vi "DroneCascadePhotos.vi"() -> ()   [LabVIEW 2017]
uses:
  <vilib>/LVH/AR Drone Toolkit/Decode NavData/Typedefs/NavData Demo.ctl
  <vilib>/LVH/AR Drone Toolkit/AR Drone.lvlib
panel:
  out "Photos Taken":dbl
  in  "Take Photos":bool
  in  "Setup Parameters":T1={"Drone IP address"="192.168.1.1", "Home IP address"="192.168.1.2", "Flight Mode"=enum."INDOOR MODE", "Mounted Hull"=enum."INDOOR HULL", "Video Camera"=2, "Max Altitude (m)"=3.0, "Max Pitch and Roll Angle (deg)"=10.0, "Max Vertical Speed (m/s)"=0.7, "Max Yaw Speed (deg/s)"=100.0} {"Video Camera" items=["Bottom Camera"=1, "Front Camera"=0, "Front in Bottom"=3, "Bottom in Front"=2]}
  out "Video Stream":picture
  out "NavData Out":T2
  out "Battery Remaining":dbl(slide) scale=0.0..100.0
  in  "Hover":bool
  in  "Take Off/Land":bool
  in  "Emergency Landing":bool
  in  "stop 2":bool
  in  "Control Cluster":T3 {"Yaw Speed" scale=-1.0..1.0; "Vertical Speed" scale=-1.0..1.0; "Pitch" scale=-1.0..1.0; "Roll" scale=-1.0..1.0}
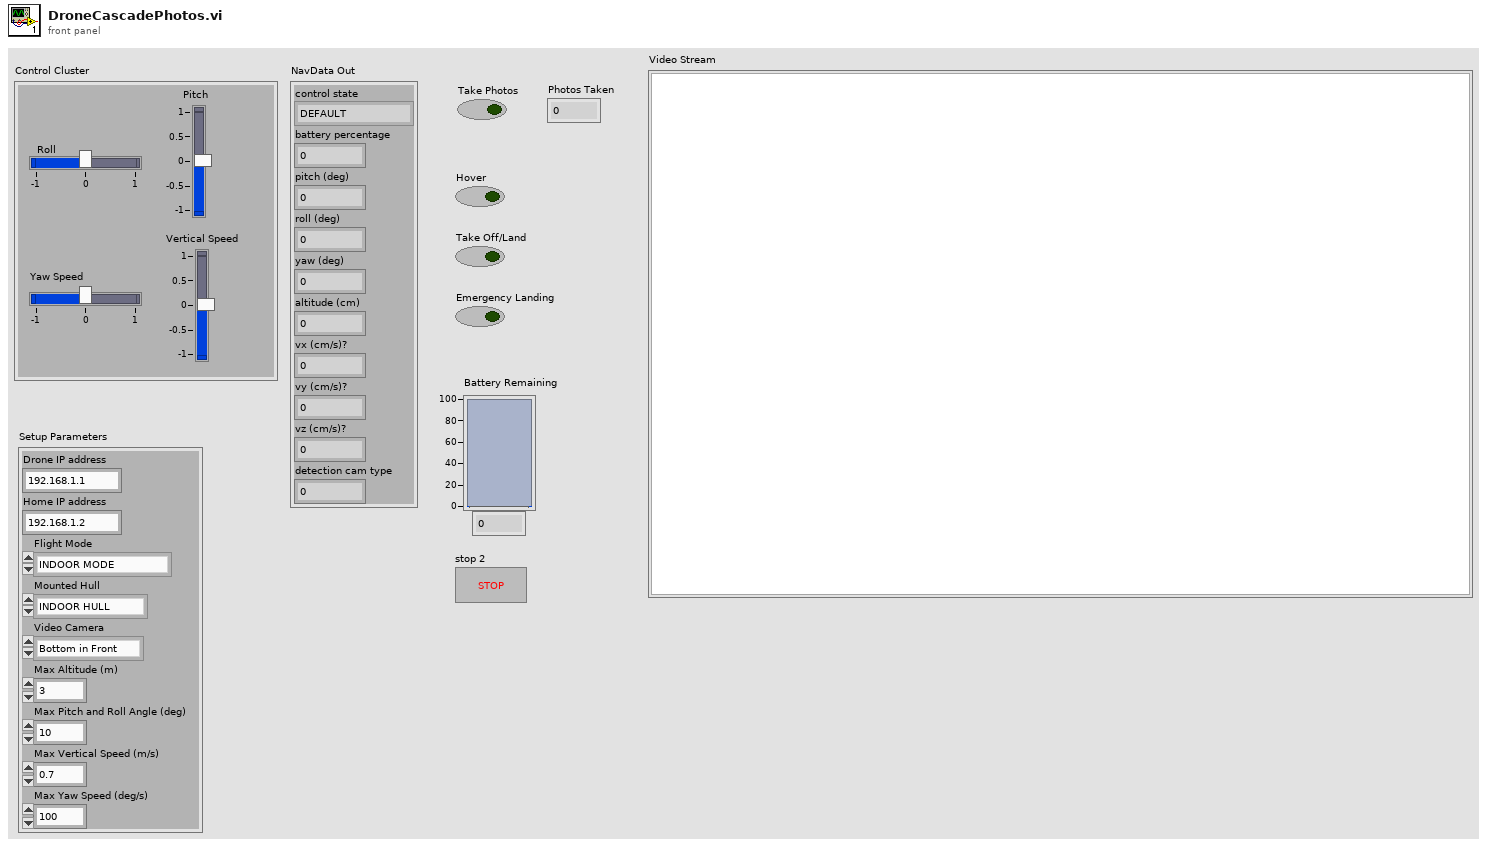
[diagram p1: front panel]
types:
  T1 = cluster{"Drone IP address":string, "Home IP address":string, "Flight Mode":enum8{"OUTDOOR MODE", "INDOOR MODE"}, "Mounted Hull":enum8{"OUTDOOR HULL", "INDOOR HULL"}, "Video Camera":u8, "Max Altitude (m)":sgl, "Max Pitch and Roll Angle (deg)":sgl, "Max Vertical Speed (m/s)":sgl, "Max Yaw Speed (deg/s)":sgl}
  T2 = typedef "AR Drone.lvlib/NavData Demo.ctl" = cluster{"control state":enum32{"DEFAULT", "INIT", "LANDING", "FLYING", "HOVERING", "TEST", "TRANS_TAKEOFF", "TRANS_GOTOFIX", "TRANS_LANDING"}, "battery percentage":u32, "pitch (deg)":sgl, "roll (deg)":sgl, "yaw (deg)":sgl, "altitude (cm)":u32, "vx (cm/s)?":sgl, "vy (cm/s)?":sgl, "vz (cm/s)?":sgl, "detection cam type":u32}
  T3 = cluster{"Roll":sgl, "Pitch":sgl, "Vertical Speed":sgl, "Yaw Speed":sgl}
  T4 = typedef "AR Drone.lvlib/AR Drone Resource.ctl" = cluster{"UDP Control Connection":refnum<k16>, "UDP NavData Connection":refnum<k16>, "UDP Video Connection (Drone 1.0)":refnum<k16>, "TCP Video Connection (Drone 2.0)":refnum<k5>, "TCP Control Port Connection":refnum<k5>, "Drone IP address":string, "Drone Command Port":u16, "Drone NavData Port":u16, "Drone Vid Stream Port":u16, "Drone TCP Control Port":u16, "Home IP address":string, "Home Command Port":u16, "Home NavData Port":u16, "Home Vid Stream Port":u16, "Drone Version":i32, "Drone Index":dbl}
  T5 = typedef "IMAQ Image.ctl" = refnum<image>
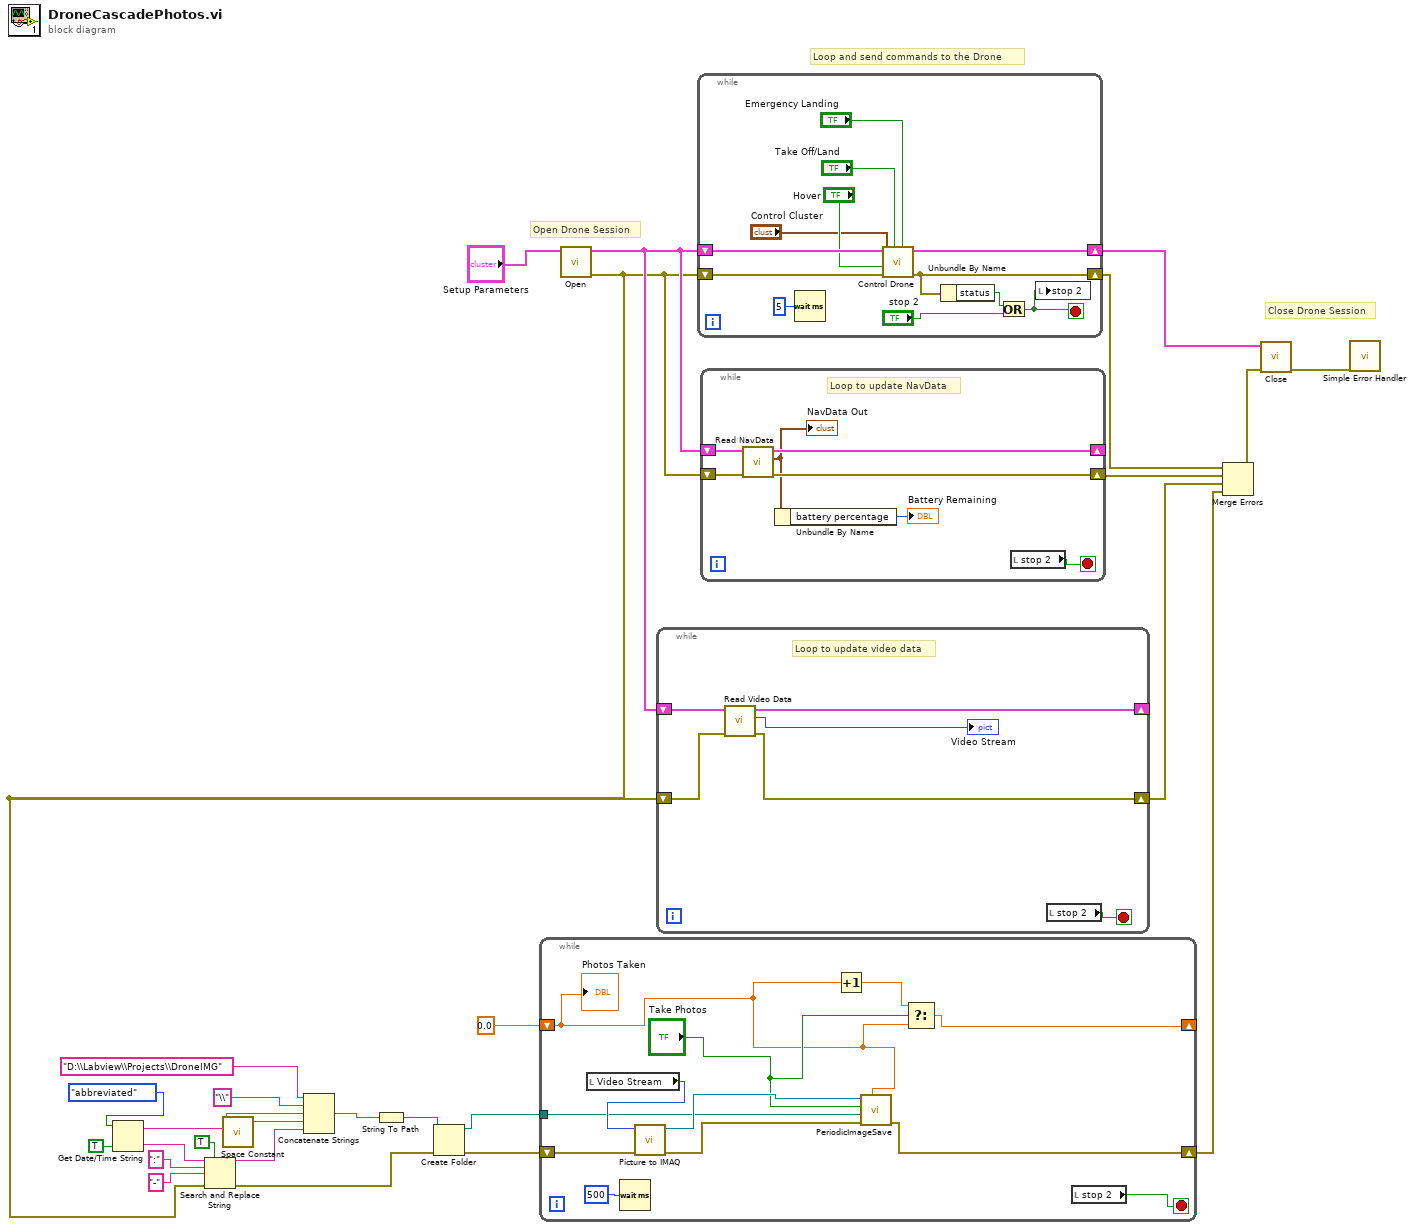
[diagram p0: block diagram]
diagram:
  # "Close Drone Session"
  # "Loop and send commands to the Drone"
  # "Open Drone Session"
  n1 = Get Date/Time String(date format (0)=enum16{"short", "long", "abbreviated"}."abbreviated", want seconds? (F)=TRUE) -> (date string=w17:string, time string=w14:string)  [unwired: 1 in]
  n2 = call <vilib>:"Space Constant.vi"() -> ("String"=w16:string)
  n3 = call <vilib>:"Open.vi"("Setup Parameters"="Setup Parameters") -> ("error out"=w4:errorcluster, "AR Drone Resource"=w25:T4)  [unwired: 9 in]
  n4 = Search and Replace String(replace all?=TRUE ("replace all? (F)"), input string=w14, search string=":" ("replace string (\"\")"), replace string="-" ("replace string (\"\")"), error in=w4) -> (result string=w15:string, error out=w5:errorcluster)  [unwired: 3 in, 2 out]
  n5 = Concatenate Strings("D:\\Labview\\Projects\\DroneIMG" ("string"), "\\" ("string"), w17, w16, w15) -> (w7:string)
  n6 = String To Path(string=w7) -> (path=w6:path)
  n7 = Create Folder(path (use dialog)=w6, error in=w5) -> (created path=w2:path, error out=w3:errorcluster)  [unwired: 1 in, 1 out]
  n8 = while {
    shift-right: [w29] -> w19
    shift-left: w3 -> [w38]
    shift-right: [w31] -> _
    shift-left: 0.0 -> [w30]
    tunnel: w2 -> [w28]
    stop <- w39 stop-if-true
    n9 = local read "Video Stream"() -> (w37:picture)
    n10 = Wait (ms)(milliseconds to wait=u32 500) -> ()  [unwired: 1 out]
    n11 = call "Picture to IMAQ.vi"("Error In"=w38, "picture"=w37) -> ("Error Out"=w35:errorcluster, "Image"=w34:T5)  [unwired: 8 in]
    n12 = Increment(x=w30) -> (x+1=w33:dbl)
    n13 = call "PeriodicImageSave.vi"("x"=w30, "error in (no error)"=w35, "in path"=w28, "Snap"="Take Photos", "Image In"=w34) -> ("error out"=w29:errorcluster)  [unwired: 5 in]
    n14 = Select(t=w33, s="Take Photos", f=w30) -> (s? t:f=w31:dbl)
    n15 = local read "stop 2"() -> (w39:bool)
    "Photos Taken" <- w30
  }
  n16 = while {
    shift-right: [w42] -> _
    shift-left: w25 -> [w44]
    shift-right: [w40] -> w20
    shift-left: w4 -> [w43]
    stop <- w45 stop-if-true
    # "Loop to update video data"
    n17 = call <vilib>:"Read Video Data.vi"("error in (no error)"=w43, "AR Drone Resource"=w44) -> ("error out"=w40:errorcluster, "Video Stream"=→"Video Stream":picture, "AR Drone Resource Out"=w42:T4)  [unwired: 7 in]
    n18 = local read "stop 2"() -> (w45:bool)
  }
  n19 = while {
    shift-right: [w52] -> w27
    shift-left: w25 -> [w56]
    shift-right: [w47] -> w22
    shift-left: w4 -> [w57]
    stop <- w46 stop-if-true
    n20 = Wait (ms)(milliseconds to wait=u32 5) -> ()  [unwired: 1 out]
    n21 = call <vilib>:"Control Drone.vi"("Emergency Landing"="Emergency Landing", "Takeoff/Land"="Take Off/Land", "error in (no error)"=w57, "Hover"="Hover", "Control Cluster"="Control Cluster", "AR Drone Resource"=w56) -> ("error out"=w47:errorcluster, "AR Drone Resource Out"=w52:T4)  [unwired: 4 in]
    n22 = Unbundle By Name(w47) -> ("status"=w49:bool)
    n23 = Or(x=w49, y="stop 2") -> (x .or. y?=w46:bool)
    n24 = local write "stop 2"(w46) -> ()
  }
  n25 = while {
    shift-right: [w62] -> _
    shift-left: w25 -> [w63]
    shift-right: [w60] -> w23
    shift-left: w4 -> [w61]
    stop <- w64 stop-if-true
    # "Loop to update NavData"
    n26 = call <vilib>:"Read NavData.vi"("error in (no error)"=w61, "AR Drone Resource"=w63) -> ("error out"=w60:errorcluster, "NavData Out"=w59:T2, "AR Drone Resource Out"=w62:T4)  [unwired: 7 in]
    "NavData Out" <- w59
    n27 = Unbundle By Name(w59) -> ("battery percentage"=→"Battery Remaining":u32)
    n28 = local read "stop 2"() -> (w64:bool)
  }
  n29 = Merge Errors(w22, w23, w20, w19) -> (w24:errorcluster)
  n30 = call <vilib>:"Close.vi"("error in (no error)"=w24, "AR Drone Resource"=w27) -> ("error out"=w26:errorcluster)  [unwired: 9 in]
  n31 = call <vilib>:"Simple Error Handler.vi"("error in (no error)"=w26) -> ()  [unwired: 4 in, 5 out]
